vi "Open.vi"(7 "Allow multiple opens?":bool, 8 "error in (no error)":errorcluster, 10 "Channel Name":tag) -> (0 "error out":errorcluster, 3 "PWM Ref Out":T1)   [LabVIEW 2021, in "PWM.lvlib"]
doc: "Opens a reference to a pulse width modulation (PWM) channel. You must open a reference before you use a PWM channel to generate PWM signals."
uses:
  <vilib>/myRIO/Instrument Drivers/Onboard IO/PWM/PWM.lvlib
  <vilib>/myRIO/Instrument Drivers/Onboard IO/PWM/typedefs/PWM Reference.ctl
  <vilib>/myRIO/Common/Instrument Driver Framework/Utilities/typedefs/myRIO Generic Hardware Reference.ctl
  <vilib>/myRIO/Common/Instrument Driver Framework/Utilities/typedefs/Hardware Version Enum.ctl
  <vilib>/myRIO/Common/Instrument Driver Framework/Utilities/typedefs/myRIO v1.0 Reference.ctl
  <vilib>/myRIO/Common/Instrument Driver Framework/Utilities/typedefs/Generic FPGA Reference.ctl
  <vilib>/myRIO/Common/Instrument Driver Framework/myRIO v1.0/PWM/typedefs/PWM Channels Enum.ctl
  <vilib>/myRIO/Instrument Drivers/Onboard IO/PWM/typedefs/PWM Configuration.ctl
  <vilib>/myRIO/Common/Instrument Driver Framework/Utilities/vis/Validate Channels.vi
  <vilib>/myRIO/Common/Instrument Driver Framework/myRIO v1.0/PWM/vis/myRIO v1.0 Reserve PWM.vi
  <vilib>/myRIO/Common/Instrument Driver Framework/roboRIO v1.0/PWM/vis/roboRIO v1.0 Reserve PWM.vi
  <vilib>/myRIO/Common/Instrument Driver Framework/ELVIS III v1.0/PWM/vis/ELVIS III v1.0 Reserve PWM.vi
  <vilib>/myRIO/Common/Instrument Driver Framework/myRIO v1.0/PWM/vis/myRIO v1.0 Build MUX Configuration PWM.vi
  <vilib>/myRIO/Common/Instrument Driver Framework/myRIO v1.0/Resource Manager/vis/myRIO v1.0 Reserve Channel List.vi
  <vilib>/myRIO/Common/Instrument Driver Framework/roboRIO v1.0/PWM/vis/roboRIO v1.0 Build MUX Configuration PWM.vi
  <vilib>/myRIO/Common/Instrument Driver Framework/roboRIO v1.0/Resource Manager/vis/roboRIO v1.0 Reserve Channel List.vi
  <vilib>/myRIO/Common/Instrument Driver Framework/ELVIS III v1.0/PWM/vis/ELVIS III v1.0 Build MUX Configuration PWM.vi
  <vilib>/myRIO/Common/Instrument Driver Framework/myRIO v1.0/Resource Manager/vis/myRIO v1.0 Create Configuration List.vi
  <vilib>/myRIO/Common/Instrument Driver Framework/myRIO v1.0/Resource Manager/vis/myRIO v1.0 Reserve Channel.vi
  <vilib>/myRIO/Common/Instrument Driver Framework/myRIO v1.0/Resource Manager/vis/myRIO v1.0 Unreserve Channel.vi
  <vilib>/myRIO/Common/Instrument Driver Framework/roboRIO v1.0/Resource Manager/vis/roboRIO v1.0 Create Configuration List.vi
  <vilib>/myRIO/Common/Instrument Driver Framework/roboRIO v1.0/Resource Manager/vis/roboRIO v1.0 Reserve Channel.vi
  <vilib>/myRIO/Common/Instrument Driver Framework/roboRIO v1.0/Resource Manager/vis/roboRIO v1.0 Unreserve Channel.vi
  <vilib>/myRIO/Common/Instrument Driver Framework/ELVIS III v1.0/Resource Manager/vis/ELVIS III v1.0 Create Configuration List.vi
  <vilib>/myRIO/Common/Instrument Driver Framework/myRIO v1.0/Resource Manager/vis/myRIO v1.0 Build Mutex Name.vi
  <vilib>/myRIO/Common/Instrument Driver Framework/roboRIO v1.0/Resource Manager/vis/roboRIO v1.0 Build Mutex Name.vi
  <vilib>/Utility/VariantDataType/GetNumericInfo.vi
  <vilib>/myRIO/Common/Instrument Driver Framework/Utilities/vis/IO Manager.vi
  <vilib>/myRIO/Common/Instrument Driver Framework/Utilities/vis/Configuration Manager.vi
  <vilib>/myRIO/Common/Instrument Driver Framework/myRIO v1.0/Resource Manager/vis/myRIO v1.0 Configure IO.vi
  <vilib>/myRIO/Common/Instrument Driver Framework/myRIO v1.0/myRIO v1.0 Close.vi
  <vilib>/myRIO/Common/Instrument Driver Framework/roboRIO v1.0/Resource Manager/vis/roboRIO v1.0 Configure IO.vi
  <vilib>/myRIO/Common/Instrument Driver Framework/ELVIS III v1.0/Resource Manager/vis/ELVIS III v1.0 Reserve Channel List.vi
  <vilib>/myRIO/Common/Instrument Driver Framework/ELVIS III v1.0/Resource Manager/vis/ELVIS III v1.0 Configure IO.vi
  <vilib>/userdefined/High Color/nirio_resource_hc.ctl
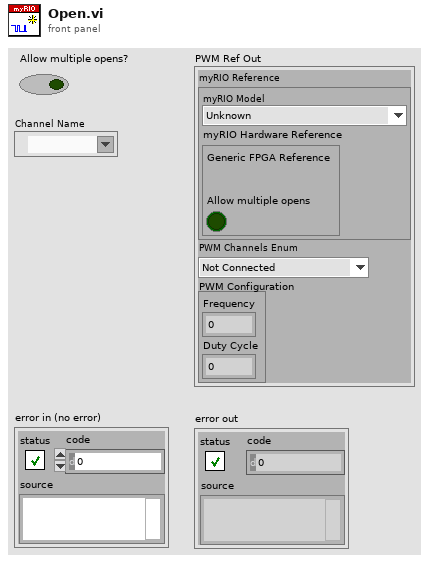
[diagram p1: front panel]
types:
  T1 = typedef "PWM.lvlib/PWM Reference.ctl" = cluster{"myRIO Reference":T2, "PWM Channels Enum":T6, "PWM Configuration":T7}
  T2 = typedef "myRIO Generic Hardware Reference.ctl" = cluster{"myRIO Model":T3, "myRIO Hardware Reference":T4}
  T3 = typedef "Hardware Version Enum.ctl" = enum16{"Unknown", "myRIO-1900", "myRIO-1950", "roboRIO", "NI ELVIS RIO CM", "ELVIS III"}
  T4 = typedef "myRIO v1.0 Reference.ctl" = cluster{"Generic FPGA Reference":T5, "Allow multiple opens":bool}
  T5 = typedef "Generic FPGA Reference.ctl" = refnum<k20>
  T6 = typedef "PWM Channels Enum.ctl" = enum16{"Not Connected", "C/PWM0", "C/PWM1", "A/PWM0", "A/PWM1", "A/PWM2", "A/PWM3", "A/PWM4", "A/PWM5", "A/PWM6", "A/PWM7", "A/PWM8", "A/PWM9", "A/PWM10", "A/PWM11", "A/PWM12", "A/PWM13", "A/PWM14", "A/PWM15", "A/PWM16", "A/PWM17", "A/PWM18", "A/PWM19", "B/PWM0", "B/PWM1", "B/PWM2", "B/PWM3", "B/PWM4", "B/PWM5", "B/PWM6", "B/PWM7", "B/PWM8", "B/PWM9", "B/PWM10", "B/PWM11", "B/PWM12", "B/PWM13", "B/PWM14", "B/PWM15", "B/PWM16", "B/PWM17", "B/PWM18", "B/PWM19", "PWM/PWM0", "PWM/PWM1", "PWM/PWM2", "PWM/PWM3", "PWM/PWM4", "PWM/PWM5", "PWM/PWM6", "PWM/PWM7", "PWM/PWM8", "PWM/PWM9"}
  T7 = typedef "PWM.lvlib/PWM Configuration.ctl" = cluster{"Frequency":dbl, "Duty Cycle":dbl}
  T8 = typedef "nirio_resource_hc.ctl" = tag
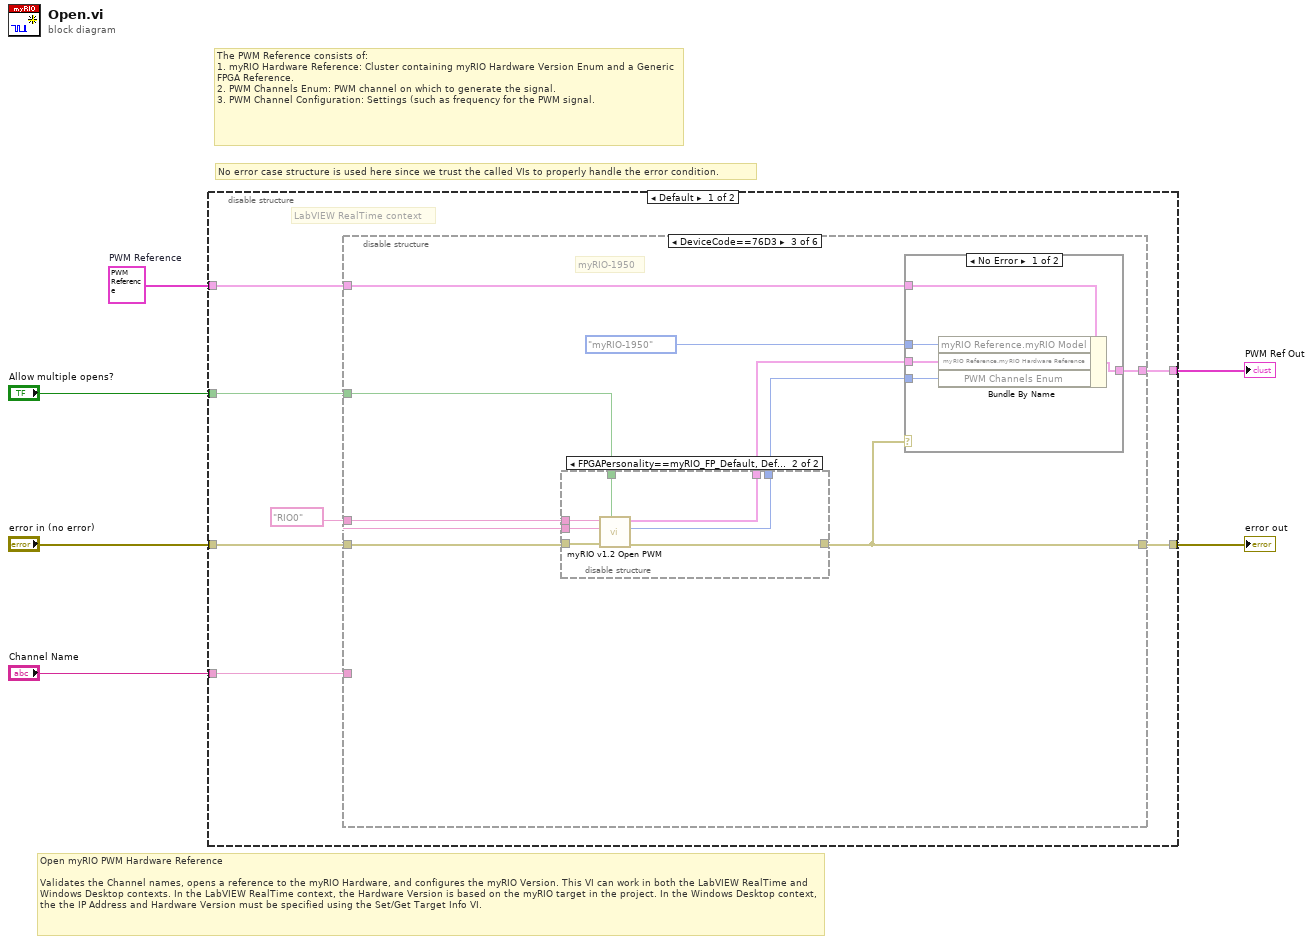
[diagram p0: block diagram]
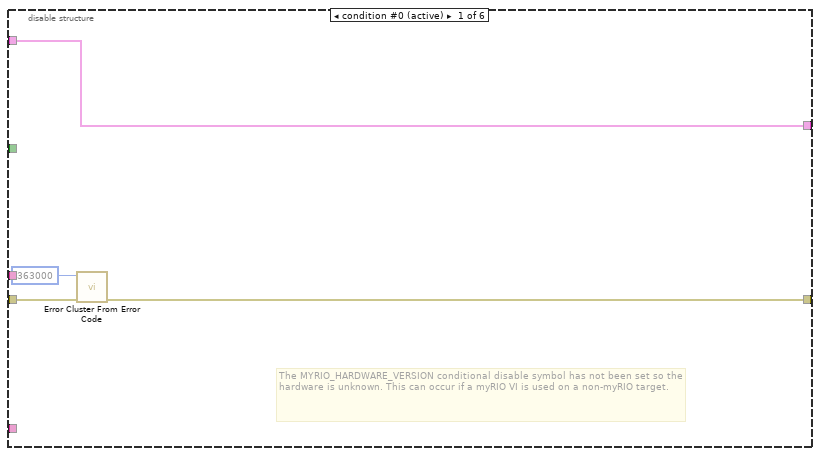
[diagram p2: hidden frame]
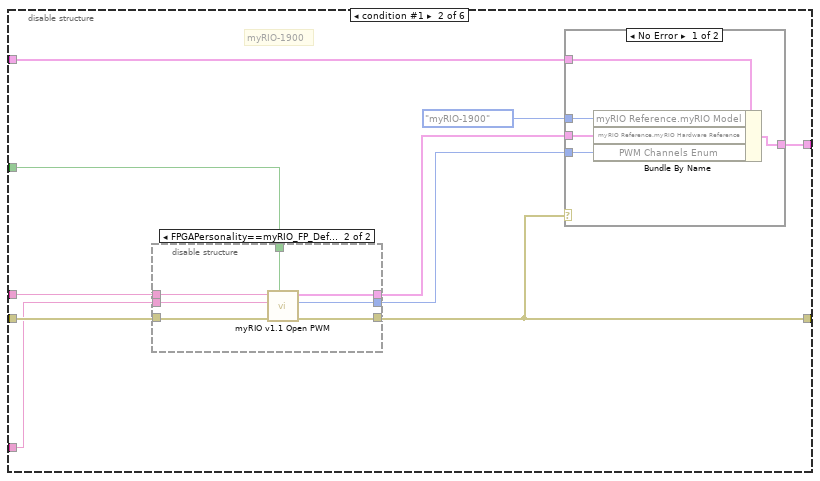
[diagram p3: hidden frame]
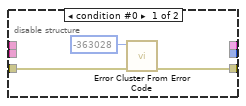
[diagram p4: hidden frame]
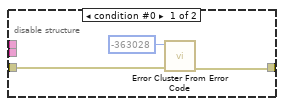
[diagram p6: hidden frame]
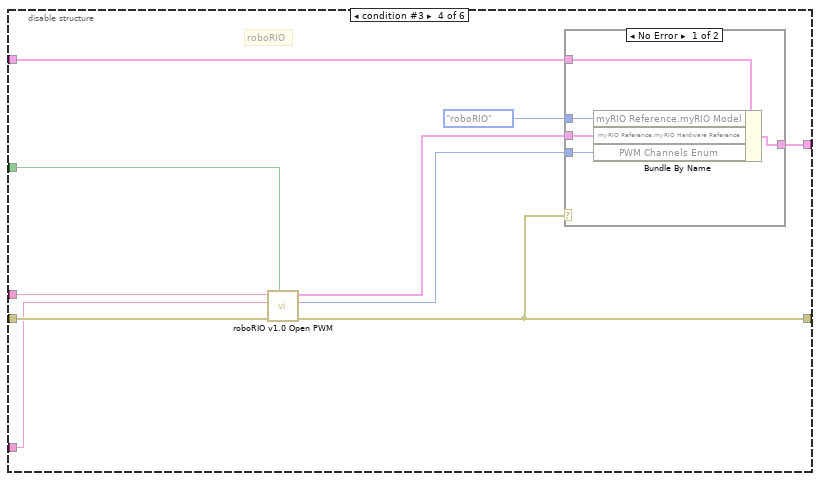
[diagram p8: hidden frame]
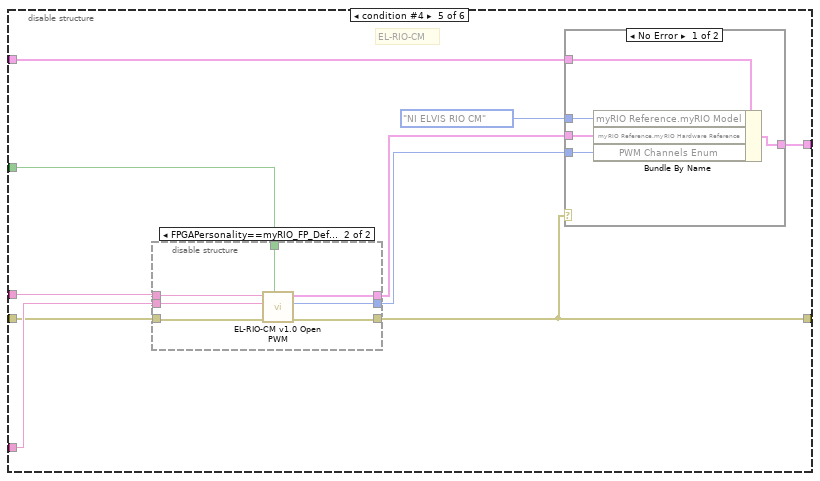
[diagram p10: hidden frame]
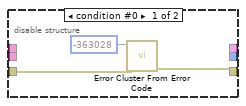
[diagram p11: hidden frame]
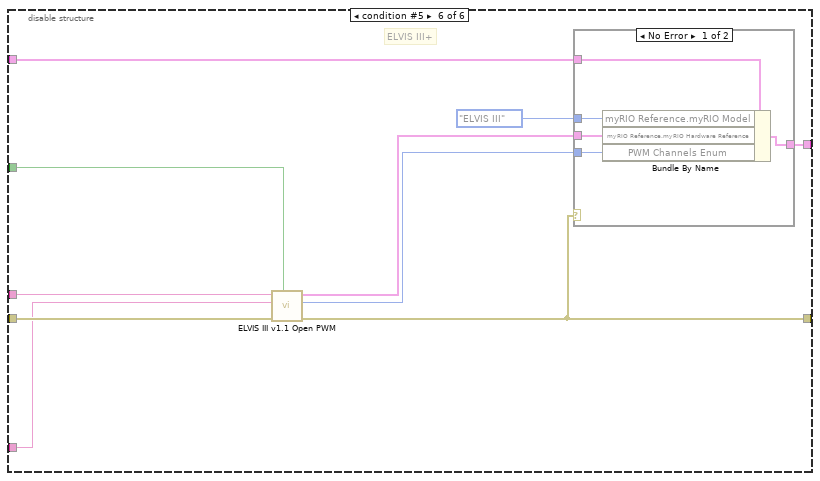
[diagram p13: hidden frame]
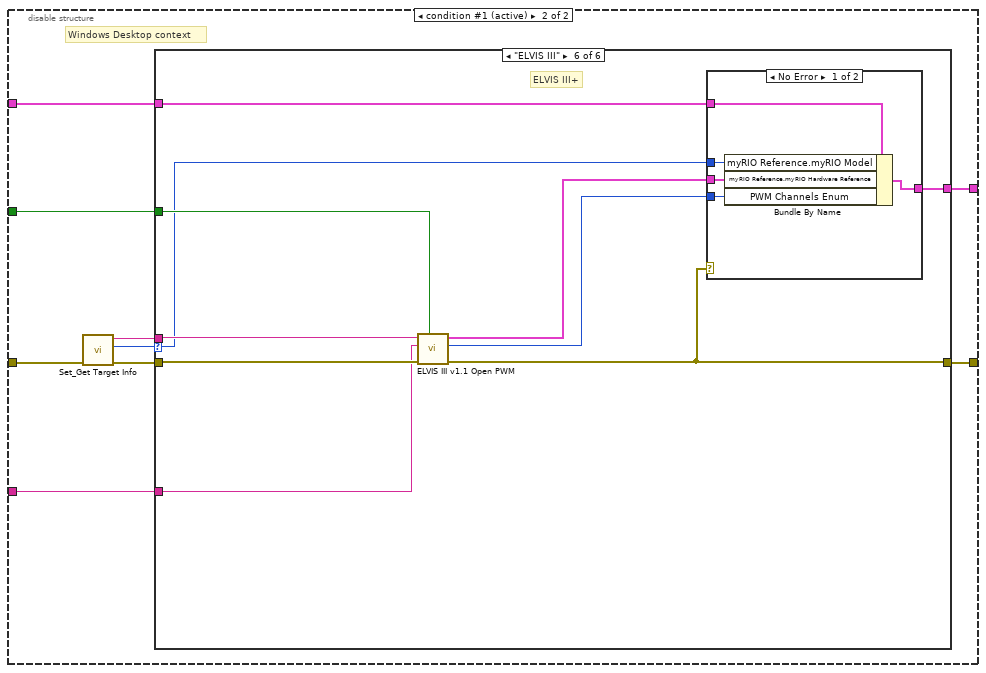
[diagram p15: hidden frame]
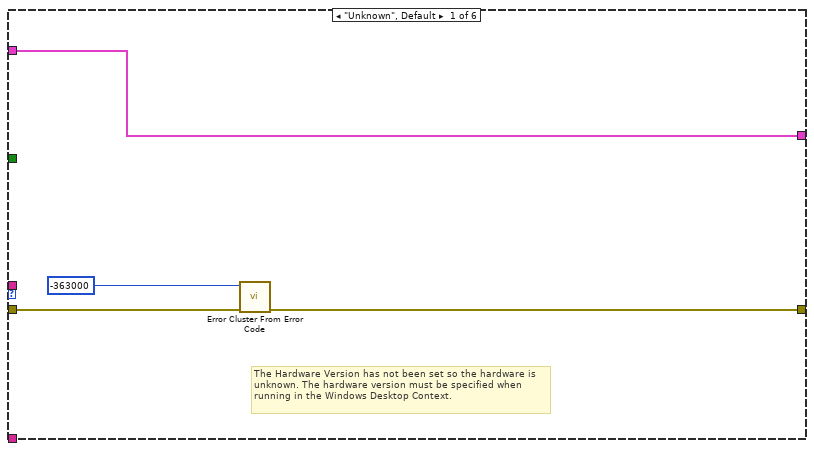
[diagram p16: hidden frame]
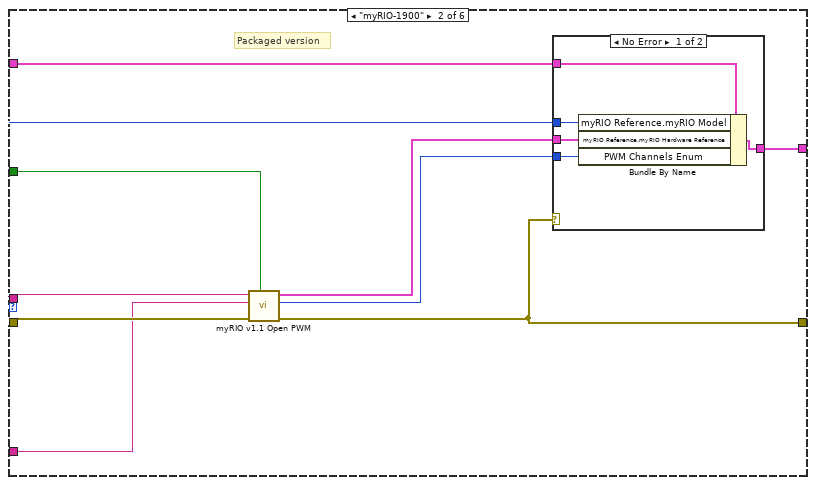
[diagram p17: hidden frame]
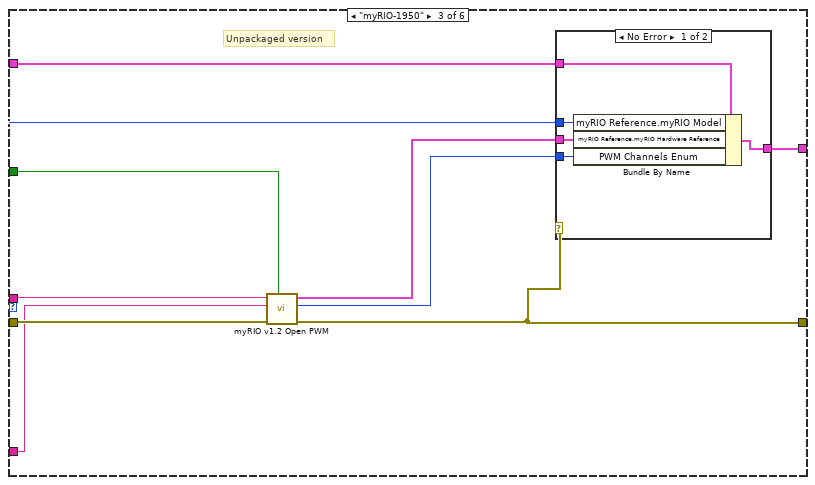
[diagram p19: hidden frame]
diagram:
  w3 = T1 {"myRIO Reference"={"myRIO Model"=enum."Unknown", "myRIO Hardware Reference"={"Generic FPGA Reference"=refnum, "Allow multiple opens"=FALSE}}, "PWM Channels Enum"=enum."Not Connected", "PWM Configuration"={"Frequency"=0.0, "Duty Cycle"=0.0}}  # PWM Reference
  # "Open myRIO PWM Hardware Reference\n\nValidates the Channel names, opens a reference to the myRIO Hardware, and configures the myRIO Version. This VI can work in both the LabVIEW RealTime and Windows Desktop contexts. In the LabVIEW RealTime context, the Hardware Version is based on the myRIO target in the project. In the Windows Desktop context, the the IP Address and Hardware Version must be specified using the Set/Get Target Info VI."
  # "No error case structure is used here since we trust the called VIs to properly handle the error condition."
  # "The PWM Reference consists of:\n1. myRIO Hardware Reference: Cluster containing myRIO Hardware Version Enum and a Generic FPGA Reference.\n2. PWM Channels Enum: PWM channel on which to generate the signal. \n3. PWM Channel Configuration: Settings (such as frequency for the PWM signal."
  n1 = disable-structure shown="Default" {
    disable-tunnel: [w13 w136] -> w6
    disable-tunnel: "error in (no error)" -> [w12 w128]
    disable-tunnel: [w11 w132] -> w2
    disable-tunnel: w3 -> [w10 w133]
    disable-tunnel: "Channel Name" -> [w9 w135]
    disable-tunnel: "Allow multiple opens?" -> [w8 w134]
    frame condition #0 {
      # "LabVIEW RealTime context"
      n2 = disable-structure shown="DeviceCode==76D3" {
        disable-tunnel: [w16 w18 w44 w70 w92 w113] -> w13
        disable-tunnel: [w14 w24 w50 w76 w94 w112] -> w11
        disable-tunnel: w12 -> [w15 w25 w51 w77 w86 w115]
        disable-tunnel: w10 -> [w14 w20 w45 w72 w93 w118]
        disable-tunnel: w9 -> [_ w23 w49 w75 w87 w114]
        disable-tunnel: w8 -> [_ w22 w47 w74 w89 w117]
        disable-tunnel: T8 "RIO0" ("Resource name") -> [_ w21 w46 w73 w88 w116]
        frame condition #0 (active) {
          # "The MYRIO_HARDWARE_VERSION conditional disable symbol has not been set so the hardware is unknown. This can occur if a myRIO VI is used on a non-myRIO target."
          n3 = call <vilib>:"Error Cluster From Error Code.vi"("error in (no error)"=w15, "error code (0)"=-363000) -> ("error out"=w16:errorcluster)  [unwired: 7 in]
        }
        frame condition #1 {
          # "myRIO-1900"
          n4 = disable-structure shown="FPGAPersonality==myRIO_FP_Default, Default" {
            disable-tunnel: [_ w37] -> w26
            disable-tunnel: w25 -> [w29 w36]
            disable-tunnel: w23 -> [_ w35]
            disable-tunnel: w22 -> [_ w34]
            disable-tunnel: w21 -> [_ w33]
            disable-tunnel: [_ w32] -> w19
            disable-tunnel: [w28 w31] -> w18
            frame condition #0 {
              n5 = call <vilib>:"Error Cluster From Error Code.vi"("error in (no error)"=w29, "error code (0)"=-363028) -> ("error out"=w28:errorcluster)  [unwired: 7 in]
            }
            frame condition #1 (active) {
              n6 = call <vilib>:"myRIO v1.1 Open PWM.vi"("Allow multiple opens?"=w34, "error in (no error)"=w36, "Channel Name"=w35, "Resource name"=w33) -> ("error out"=w31:errorcluster, "PWM Channel"=w32:T6, "myRIO Ref Out"=w37:T4)  [unwired: 5 in]
            }
          }
          n7 = case shown="No Error" w18 {
            tunnel: Hardware_Version_Enum."myRIO-1900" ("Hardware Version") -> [w42 _]
            tunnel: w26 -> [w38 _]
            tunnel: [w41 w43] -> w24
            tunnel: w19 -> [w40 _]
            tunnel: w20 -> [w39 w43]
            frame No Error {
              n8 = Bundle By Name(cluster=w39, "myRIO Reference.myRIO Model"=w42, "myRIO Reference.myRIO Hardware Reference"=w38, "PWM Channels Enum"=w40) -> (w41:T1)
            }
            frame Error {
            }
          }
        }
        frame condition #2 {
          # "myRIO-1950"
          n9 = disable-structure shown="FPGAPersonality==myRIO_FP_Default, Default" {
            disable-tunnel: [_ w63] -> w52
            disable-tunnel: w51 -> [w55 w62]
            disable-tunnel: w49 -> [_ w61]
            disable-tunnel: [_ w60] -> w48
            disable-tunnel: w47 -> [_ w59]
            disable-tunnel: w46 -> [_ w58]
            disable-tunnel: [w54 w57] -> w44
            frame condition #0 {
              n10 = call <vilib>:"Error Cluster From Error Code.vi"("error in (no error)"=w55, "error code (0)"=-363028) -> ("error out"=w54:errorcluster)  [unwired: 7 in]
            }
            frame condition #1 (active) {
              n11 = call <vilib>:"myRIO v1.2 Open PWM.vi"("Allow multiple opens?"=w59, "error in (no error)"=w62, "Channel Name"=w61, "Resource name"=w58) -> ("error out"=w57:errorcluster, "PWM Channel"=w60:T6, "myRIO Ref Out"=w63:T4)  [unwired: 5 in]
            }
          }
          n12 = case shown="No Error" w44 {
            tunnel: Hardware_Version_Enum."myRIO-1950" ("Hardware Version") -> [w68 _]
            tunnel: w52 -> [w67 _]
            tunnel: [w66 w69] -> w50
            tunnel: w48 -> [w65 _]
            tunnel: w45 -> [w64 w69]
            frame No Error {
              n13 = Bundle By Name(cluster=w64, "myRIO Reference.myRIO Model"=w68, "myRIO Reference.myRIO Hardware Reference"=w67, "PWM Channels Enum"=w65) -> (w66:T1)
            }
            frame Error {
            }
          }
        }
        frame condition #3 {
          # "roboRIO"
          n14 = call <vilib>:"roboRIO v1.0 Open PWM.vi"("Allow multiple opens?"=w74, "error in (no error)"=w77, "Channel Name"=w75, "Resource name"=w73) -> ("error out"=w70:errorcluster, "PWM Channel"=w71:T6, "myRIO Ref Out"=w78:T4)  [unwired: 5 in]
          n15 = case shown="No Error" w70 {
            tunnel: Hardware_Version_Enum."roboRIO" ("Hardware Version") -> [w84 _]
            tunnel: w78 -> [w80 _]
            tunnel: [w83 w85] -> w76
            tunnel: w71 -> [w82 _]
            tunnel: w72 -> [w81 w85]
            frame No Error {
              n16 = Bundle By Name(cluster=w81, "myRIO Reference.myRIO Model"=w84, "myRIO Reference.myRIO Hardware Reference"=w80, "PWM Channels Enum"=w82) -> (w83:T1)
            }
            frame Error {
            }
          }
        }
        frame condition #4 {
          # "EL-RIO-CM"
          n17 = disable-structure shown="FPGAPersonality==myRIO_FP_Default, Default" {
            disable-tunnel: [_ w103] -> w90
            disable-tunnel: w86 -> [w97 w100]
            disable-tunnel: w88 -> [_ w102]
            disable-tunnel: w87 -> [_ w101]
            disable-tunnel: [_ w104] -> w91
            disable-tunnel: w89 -> [_ w99]
            disable-tunnel: [w96 w105] -> w92
            frame condition #0 {
              n18 = call <vilib>:"Error Cluster From Error Code.vi"("error in (no error)"=w97, "error code (0)"=-363028) -> ("error out"=w96:errorcluster)  [unwired: 7 in]
            }
            frame condition #1 (active) {
              n19 = call <vilib>:"EL-RIO-CM v1.0 Open PWM.vi"("Allow multiple opens?"=w99, "error in (no error)"=w100, "Channel Name"=w101, "Resource name"=w102) -> ("error out"=w105:errorcluster, "PWM Channel"=w104:T6, "myRIO Ref Out"=w103:T4)  [unwired: 5 in]
            }
          }
          n20 = case shown="No Error" w92 {
            tunnel: Hardware_Version_Enum."NI ELVIS RIO CM" ("Hardware Version") -> [w110 _]
            tunnel: w90 -> [w106 _]
            tunnel: [w109 w111] -> w94
            tunnel: w91 -> [w108 _]
            tunnel: w93 -> [w107 w111]
            frame No Error {
              n21 = Bundle By Name(cluster=w107, "myRIO Reference.myRIO Model"=w110, "myRIO Reference.myRIO Hardware Reference"=w106, "PWM Channels Enum"=w108) -> (w109:T1)
            }
            frame Error {
            }
          }
        }
        frame condition #5 {
          # "ELVIS III+"
          n22 = call <vilib>:"ELVIS III v1.1 Open PWM.vi"("Allow multiple opens?"=w117, "error in (no error)"=w115, "Channel Name"=w114, "Resource name"=w116) -> ("error out"=w113:errorcluster, "PWM Channel"=w120:T6, "myRIO Ref Out"=w119:T4)  [unwired: 5 in]
          n23 = case shown="No Error" w113 {
            tunnel: Hardware_Version_Enum."ELVIS III" ("Hardware Version") -> [w126 _]
            tunnel: w119 -> [w122 _]
            tunnel: [w125 w127] -> w112
            tunnel: w120 -> [w124 _]
            tunnel: w118 -> [w123 w127]
            frame No Error {
              n24 = Bundle By Name(cluster=w123, "myRIO Reference.myRIO Model"=w126, "myRIO Reference.myRIO Hardware Reference"=w122, "PWM Channels Enum"=w124) -> (w125:T1)
            }
            frame Error {
            }
          }
        }
      }
    }
    frame condition #1 (active) {
      # "Windows Desktop context"
      n25 = call <vilib>:"Set_Get Target Info.vi"("error in (no error)"=w128) -> ("error out"=w129:errorcluster, "Hardware Version"=w130:T3, "IP Address"=w131:string)  [unwired: 8 in]
      n26 = case shown="\"ELVIS III\"" w130 {
        selector: w130 -> [_ w142 w158 w174 w190 w209]
        tunnel: [w139 w141 w157 w173 w189 w206] -> w136
        tunnel: w131 -> [_ w149 w165 w181 w197 w210]
        tunnel: w129 -> [w138 w148 w164 w180 w196 w208]
        tunnel: [w137 w147 w163 w179 w195 w205] -> w132
        tunnel: w135 -> [_ w146 w162 w178 w194 w207]
        tunnel: w134 -> [_ w145 w160 w176 w192 w211]
        tunnel: w133 -> [w137 w143 w159 w175 w191 w212]
        frame "Unknown", Default {
          # "The Hardware Version has not been set so the hardware is unknown. The hardware version must be specified when running in the Windows Desktop Context."
          n27 = call <vilib>:"Error Cluster From Error Code.vi"("error in (no error)"=w138, "error code (0)"=-363000) -> ("error out"=w139:errorcluster)  [unwired: 7 in]
        }
        frame "myRIO-1900" {
          # "Packaged version"
          n28 = call <vilib>:"myRIO v1.1 Open PWM.vi"("Allow multiple opens?"=w145, "error in (no error)"=w148, "Channel Name"=w146, "Resource name"=w149) -> ("error out"=w141:errorcluster, "PWM Channel"=w144:T6, "myRIO Ref Out"=w150:T4)  [unwired: 5 in]
          n29 = case shown="No Error" w141 {
            tunnel: w142 -> [w155 _]
            tunnel: w150 -> [w154 _]
            tunnel: [w153 w156] -> w147
            tunnel: w144 -> [w152 _]
            tunnel: w143 -> [w151 w156]
            frame No Error {
              n30 = Bundle By Name(cluster=w151, "myRIO Reference.myRIO Model"=w155, "myRIO Reference.myRIO Hardware Reference"=w154, "PWM Channels Enum"=w152) -> (w153:T1)
            }
            frame Error {
            }
          }
        }
        frame "myRIO-1950" {
          # "Unpackaged version"
          n31 = call <vilib>:"myRIO v1.2 Open PWM.vi"("Allow multiple opens?"=w160, "error in (no error)"=w164, "Channel Name"=w162, "Resource name"=w165) -> ("error out"=w157:errorcluster, "PWM Channel"=w161:T6, "myRIO Ref Out"=w166:T4)  [unwired: 5 in]
          n32 = case shown="No Error" w157 {
            tunnel: w158 -> [w171 _]
            tunnel: w166 -> [w170 _]
            tunnel: [w169 w172] -> w163
            tunnel: w161 -> [w168 _]
            tunnel: w159 -> [w167 w172]
            frame No Error {
              n33 = Bundle By Name(cluster=w167, "myRIO Reference.myRIO Model"=w171, "myRIO Reference.myRIO Hardware Reference"=w170, "PWM Channels Enum"=w168) -> (w169:T1)
            }
            frame Error {
            }
          }
        }
        frame "roboRIO" {
          # "Unpackaged version"
          n34 = call <vilib>:"roboRIO v1.0 Open PWM.vi"("Allow multiple opens?"=w176, "error in (no error)"=w180, "Channel Name"=w178, "Resource name"=w181) -> ("error out"=w173:errorcluster, "PWM Channel"=w177:T6, "myRIO Ref Out"=w182:T4)  [unwired: 5 in]
          n35 = case shown="No Error" w173 {
            tunnel: w174 -> [w187 _]
            tunnel: w182 -> [w186 _]
            tunnel: [w185 w188] -> w179
            tunnel: w177 -> [w184 _]
            tunnel: w175 -> [w183 w188]
            frame No Error {
              n36 = Bundle By Name(cluster=w183, "myRIO Reference.myRIO Model"=w187, "myRIO Reference.myRIO Hardware Reference"=w186, "PWM Channels Enum"=w184) -> (w185:T1)
            }
            frame Error {
            }
          }
        }
        frame "NI ELVIS RIO CM" {
          # "EL-RIO-CM"
          n37 = call <vilib>:"EL-RIO-CM v1.0 Open PWM.vi"("Allow multiple opens?"=w192, "error in (no error)"=w196, "Channel Name"=w194, "Resource name"=w197) -> ("error out"=w189:errorcluster, "PWM Channel"=w193:T6, "myRIO Ref Out"=w198:T4)  [unwired: 5 in]
          n38 = case shown="No Error" w189 {
            tunnel: w190 -> [w203 _]
            tunnel: w198 -> [w202 _]
            tunnel: [w201 w204] -> w195
            tunnel: w193 -> [w200 _]
            tunnel: w191 -> [w199 w204]
            frame No Error {
              n39 = Bundle By Name(cluster=w199, "myRIO Reference.myRIO Model"=w203, "myRIO Reference.myRIO Hardware Reference"=w202, "PWM Channels Enum"=w200) -> (w201:T1)
            }
            frame Error {
            }
          }
        }
        frame "ELVIS III" {
          # "ELVIS III+"
          n40 = call <vilib>:"ELVIS III v1.1 Open PWM.vi"("Allow multiple opens?"=w211, "error in (no error)"=w208, "Channel Name"=w207, "Resource name"=w210) -> ("error out"=w206:errorcluster, "PWM Channel"=w213:T6, "myRIO Ref Out"=w214:T4)  [unwired: 5 in]
          n41 = case shown="No Error" w206 {
            tunnel: w209 -> [w219 _]
            tunnel: w214 -> [w218 _]
            tunnel: [w217 w220] -> w205
            tunnel: w213 -> [w216 _]
            tunnel: w212 -> [w215 w220]
            frame No Error {
              n42 = Bundle By Name(cluster=w215, "myRIO Reference.myRIO Model"=w219, "myRIO Reference.myRIO Hardware Reference"=w218, "PWM Channels Enum"=w216) -> (w217:T1)
            }
            frame Error {
            }
          }
        }
      }
    }
  }
  "PWM Ref Out" <- w2
  "error out" <- w6
